vi "KepcoDCPwr Self-Test.vi"(0 "VISA Session":refnum<visa-resource-name>, 5 "Model In":string, 7 "channel name (\"\")":string="\"\"", 11 "error in (no error)":errorcluster {"code" format="%.0x"}) -> (4 "VISA Session Out":refnum<visa-resource-name>, 6 "Model Out":string, 8 "channel name out (\"\")":string="\"\"" caption="channel name Out (\"\")", 10 "self test result":i32 format="%.0x", 14 "self-test message":string, 15 "error out":errorcluster {"code" format="%.0x"})   [LabVIEW 2010]
doc: "This VI runs the instrument's self test routine and returns the test result(s)."
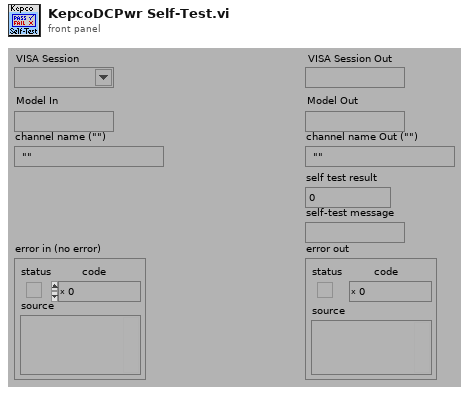
[diagram p1: front panel]
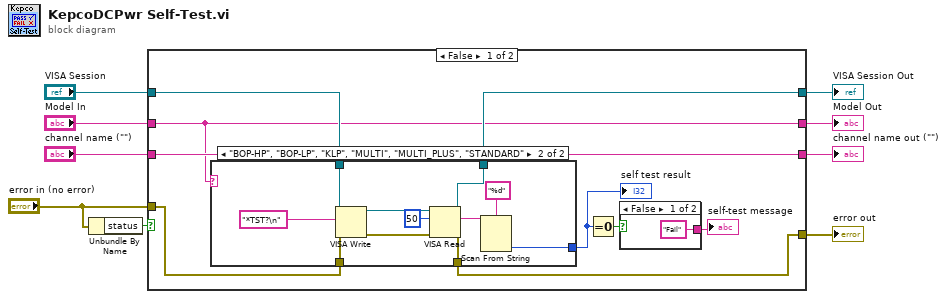
[diagram p0: block diagram]
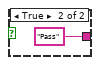
[diagram p2: hidden frame]
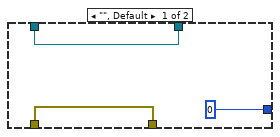
[diagram p3: hidden frame]
diagram:
  n1 = Unbundle By Name("error in (no error)") -> ("status"=w8:bool)
  n2 = case shown="False" w8 {
    tunnel: [w15 w38] -> w9
    tunnel: "error in (no error)" -> [w14 w38]
    tunnel: [w16 w37] -> w1
    tunnel: "VISA Session" -> [w17 w37]
    tunnel: [w13 w36] -> w2
    tunnel: "Model In" -> [w13 w36]
    tunnel: [w18 w35] -> w3
    tunnel: "channel name (\"\")" -> [w18 w35]
    frame False {
      n3 = case shown="\"BOP-HP\", \"BOP-LP\", \"KLP\", \"MULTI\", \"MULTI_PLUS\", \"STANDARD\"" w13 {
        tunnel: [w21 w28] -> w16
        tunnel: w17 -> [w21 w33]
        tunnel: w14 -> [w23 w32]
        tunnel: [w23 w29] -> w15
        tunnel: [0 w26] -> w12
        frame "", Default {
        }
        frame "BOP-HP", "BOP-LP", "KLP", "MULTI", "MULTI_PLUS", "STANDARD" {
          n4 = VISA Write(VISA resource name=w33, write buffer="*TST?\n", error in (no error)=w32) -> (VISA resource name out=w30:refnum<visa-resource-name>, error out=w31:errorcluster)  [unwired: 1 out]
          n5 = VISA Read(VISA resource name=w30, byte count=u32 50 ("byte count (0)"), error in (no error)=w31) -> (VISA resource name out=w28:refnum<visa-resource-name>, read buffer=w27:string, error out=w29:errorcluster)  [unwired: 1 out]
          n6 = Scan From String(format string="%d", input string=w27) -> (output 1=w26:i32)  [unwired: 3 in, 3 out]
        }
      }
      "self test result" <- w12
      n7 = Equal To 0?(x=w12) -> (x = 0?=w11:bool)
      n8 = case shown="False" w11 {
        tunnel: ["Fail" "Pass"] -> w10
        frame False {
        }
        frame True {
        }
      }
      "self-test message" <- w10
    }
    frame True {
    }
  }
  "error out" <- w9
  "channel name out (\"\")" <- w3
  "Model Out" <- w2
  "VISA Session Out" <- w1
